vi "Main Engine.vi"() -> ()   [LabVIEW 2014, in "Sample QSM.lvlib"]
uses:
  Sample QSM.lvlib
  Typedefs/Queue Commands.ctl
  Typedefs/Main Cluster.ctl
panel:
  out "Status":string
  in  "Stop Button":bool
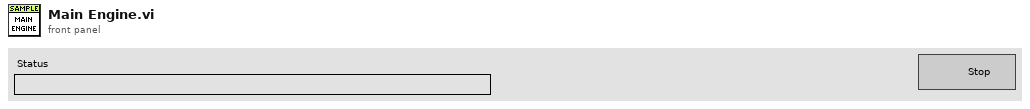
[diagram p1: front panel]
types:
  T1 = typedef "Sample QSM.lvlib/Queue Commands.ctl" = enum16{"Create", "Enqueue", "Enqueue N", "Enstack", "Dequeue", "Flush", "Release"}
  T2 = typedef "Sample QSM.lvlib/Main Cluster.ctl" = cluster{string}
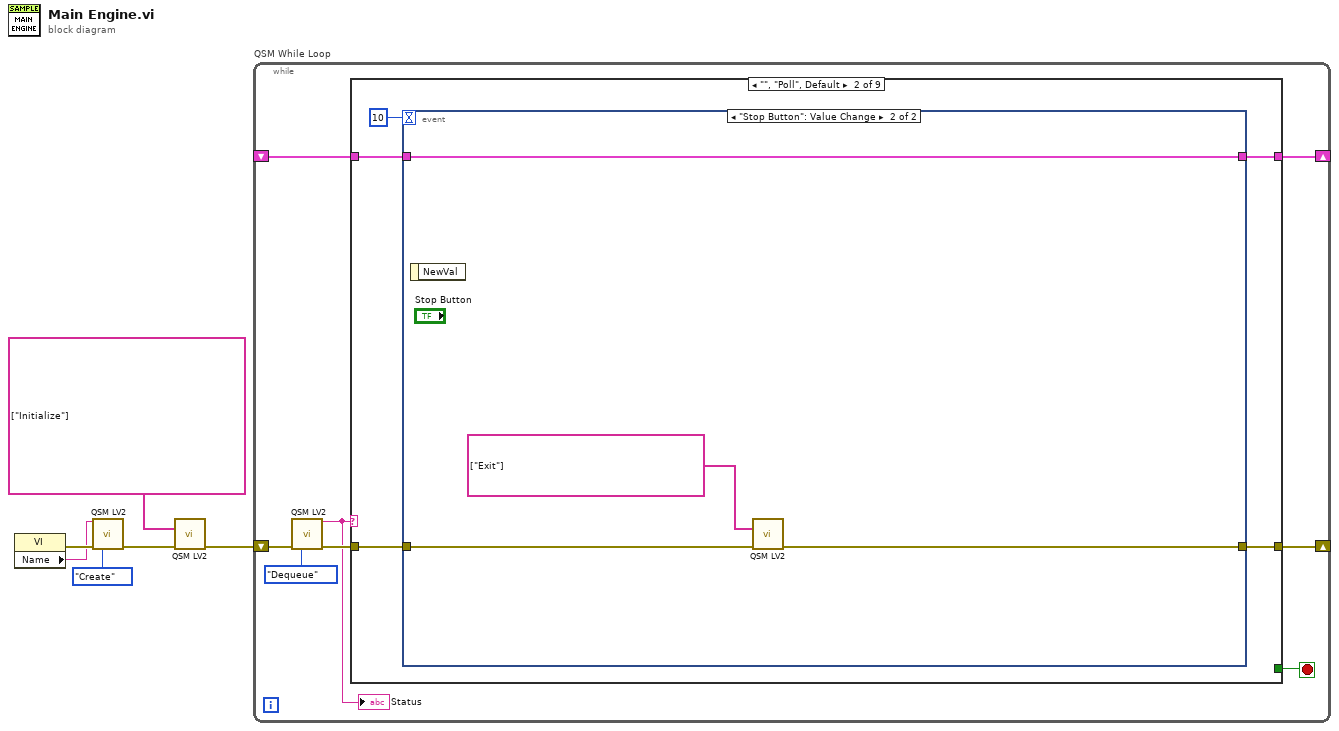
[diagram p0: block diagram]
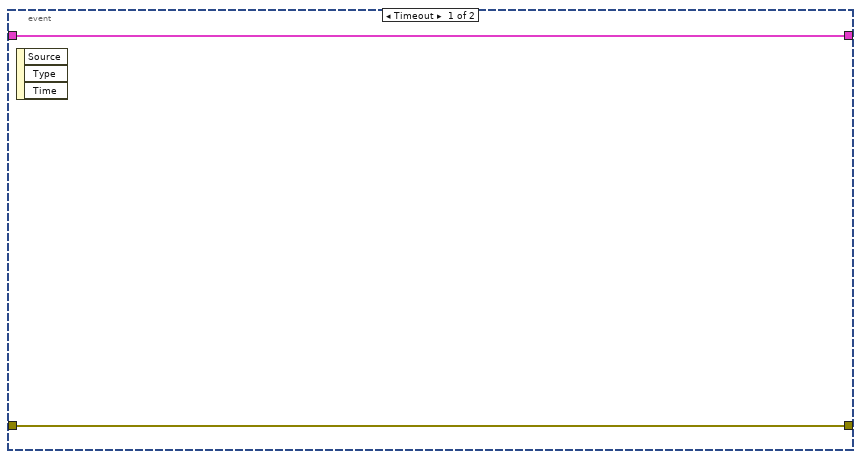
[diagram p3: hidden frame]
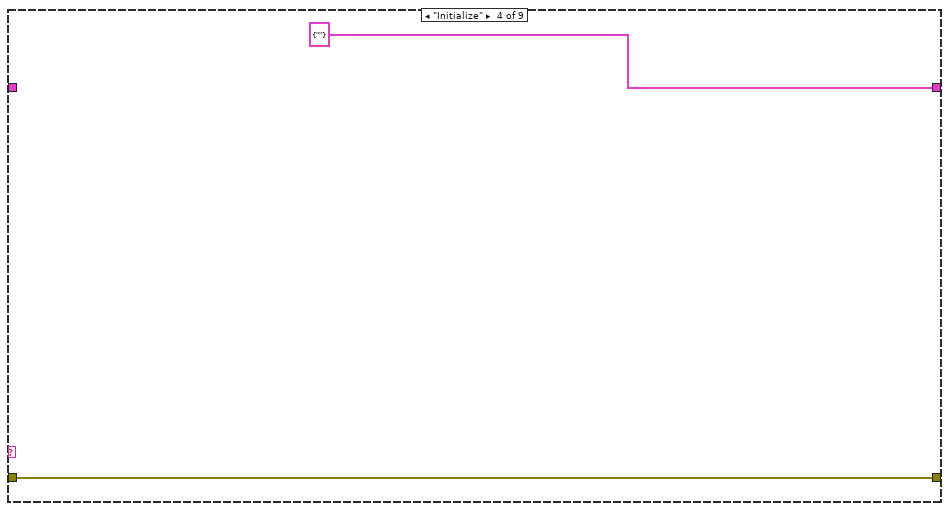
[diagram p5: hidden frame]
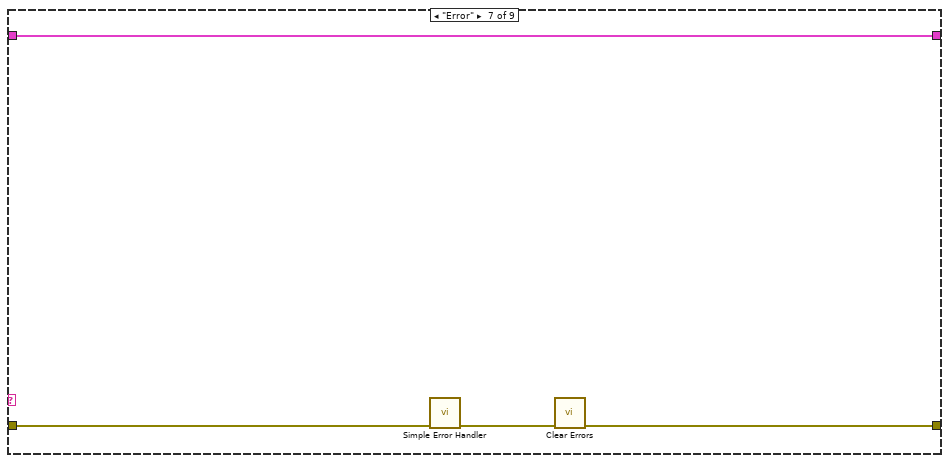
[diagram p8: hidden frame]
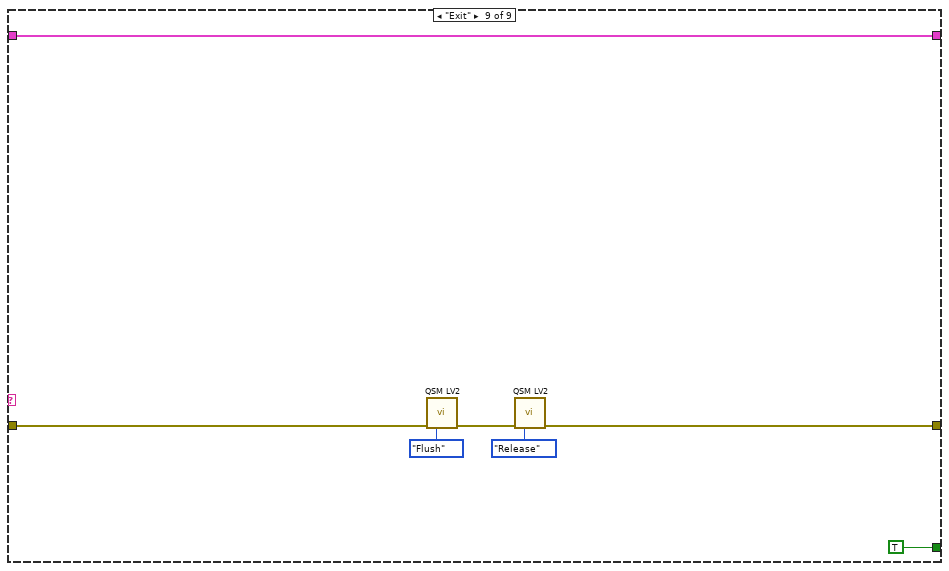
[diagram p10: hidden frame]
diagram:
  n1 = property class="VI"() -> (error out=w6:errorcluster, "Name"=w5:string)  [unwired: 2 in, 1 out]
  n2 = call "QSM LV2.vi"("Queue Name"=w5, "Error In"=w6, "Command"=Queue_Commands."Create") -> ("Error Out"=w3:errorcluster)  [unwired: 11 in, 1 out]
  n3 = call "QSM LV2.vi"("Enqueue N"=string[] ["Initialize"], "Error In"=w3) -> ("Error Out"=w2:errorcluster)  [unwired: 12 in, 1 out]
  n4 = while "QSM While Loop" {
    shift-right: [w11] -> _
    shift-left: w2 -> [w14]
    shift-right: [w9] -> _
    shift-left: _ -> [w8]
    stop <- w10 stop-if-true
    n5 = call "QSM LV2.vi"("Error In"=w14, "Command"=Queue_Commands."Dequeue") -> ("Dequeue"=w7:string, "Error Out"=w12:errorcluster)  [unwired: 12 in]
    "Status" <- w7
    n6 = case "QSM Case Structure" shown="\"\", \"Poll\", Default" w7 {
      tunnel: w12 -> [w16 w19 w29 w31 w33 w35 w39 w41 w44]
      tunnel: [w16 w20 w29 w31 w33 w35 w36 w41 w43] -> w11
      tunnel: [_ _ _ _ _ _ _ _ TRUE] -> w10
      tunnel: [w15 w17 w28 T2 {""} w32 w34 w38 w40 w42] -> w9
      tunnel: w8 -> [w15 w18 w28 _ w32 w34 w38 w40 w42]
      frame "/**** Poll ****/" {
      }
      frame "", "Poll", Default {
        n7 = event shown="[1] \"Stop Button\": Value Change" {
          selector: _ -> [_ _]
          dyn-events: _ -> [_ _]
          timeout: 10 -> [_ _]
          tunnel: [w23 w26] -> w20
          tunnel: w19 -> [w23 w27]
          tunnel: w18 -> [w22 w25]
          tunnel: [w22 w25] -> w17
          event Timeout {
            n8 = event-data() -> ()  [unwired: 1 in, 3 out]
          }
          event "Stop Button": Value Change {
            n9 = event-data() -> ()  [unwired: 1 in, 1 out]
            n10 = call "QSM LV2.vi"("Enqueue N"=string[] ["Exit"], "Error In"=w27) -> ("Error Out"=w26:errorcluster)  [unwired: 12 in, 1 out]
          }
        }
      }
      frame "/**** Initialize ****/" {
      }
      frame "Initialize" {
      }
      frame "/*** Custom Case Splitter ***/" {
      }
      frame "/*** Error Handler ***/" {
      }
      frame "Error" {
        n11 = call <vilib>:"Simple Error Handler.vi"("error in (no error)"=w39) -> ("error out"=w37:errorcluster)  [unwired: 4 in, 4 out]
        n12 = call <vilib>:"Clear Errors.vi"("error in (no error)"=w37) -> ("error out"=w36:errorcluster)  [unwired: 5 in, 1 out]
      }
      frame "/**** Exit ****/" {
      }
      frame "Exit" {
        n13 = call "QSM LV2.vi"("Error In"=w44, "Command"=Queue_Commands."Flush") -> ("Error Out"=w45:errorcluster)  [unwired: 12 in, 1 out]
        n14 = call "QSM LV2.vi"("Error In"=w45, "Command"=Queue_Commands."Release") -> ("Error Out"=w43:errorcluster)  [unwired: 12 in, 1 out]
      }
    }
  }
